vi "readcsv.vi"(8 "error in":errorcluster) -> (0 "error out":errorcluster, 3 "Zone Setup Array":cluster{"Zone Selector":string, "Timing":dbl}[](array[cluster]))   [LabVIEW 2015]
uses:
  <vilib>/Utility/file.llb/Read Delimited Spreadsheet (string).vi
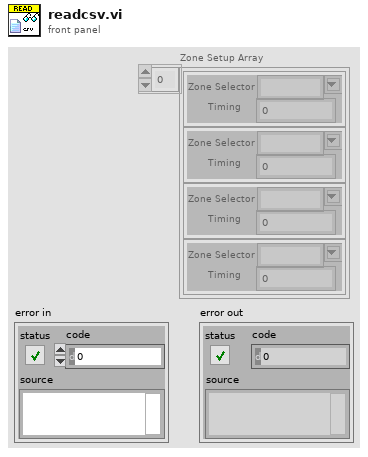
[diagram p1: front panel]
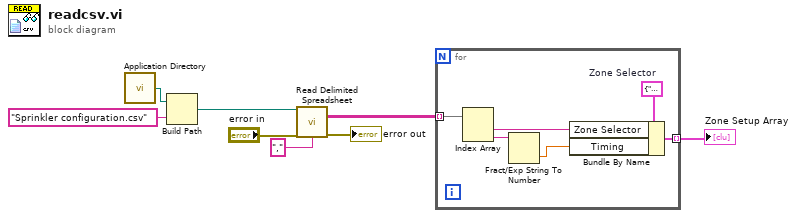
[diagram p0: block diagram]
diagram:
  n1 = call <vilib>:"Application Directory.vi"() -> ("Application Directory"=w5:path)
  n2 = Build Path(base path=w5, name or relative path="Sprinkler configuration.csv") -> (appended path=w7:path)
  n3 = call-poly <vilib>:"Read Delimited Spreadsheet.vi"("file path (dialog if empty)"=w7, "error in (no error)"="error in", "delimiter (\\t)"="," ("delimiter (\\t)")) -> ("all rows"=w3:string[][], "error out"=→"error out":errorcluster)  [unwired: 7 in, 4 out]
  n4 = for {
    tunnel: w3 -> [w14] mode=indexing
    tunnel: [w9] -> w2 mode=indexing
    w12 = cluster{"Zone Selector":string, "Timing":dbl} {"Zone Selector"="", "Timing"=0.0}  # Zone Selector
    n5 = Index Array(array=w14) -> (element #1=w10:string, element #2=w13:string)  [unwired: 2 in]
    n6 = Fract/Exp String To Number(string=w13) -> (number=w11:dbl)  [unwired: 3 in, 1 out]
    n7 = Bundle By Name(cluster=w12, "Zone Selector"=w10, "Timing"=w11) -> (w9:cluster{"Zone Selector":string, "Timing":dbl})
  }
  "Zone Setup Array" <- w2
